vi "Streaming Xcvr (FPGA) Rx.vi"() -> ()   [LabVIEW 2016]
doc: "Acquires data from the Rx ports and streams the data to the host while receiving data from the host and generating the resulting waveform at the Tx ports of the NI USRP-294x/295x device. Use this VI as a template for the Simple NI-USRP Streaming sample project."
uses:
  <instrlib>/_niInstr/Register Bus/v1/FPGA/Public/Read Cmd Data.ctl
  SubVIs/Tx Parameters.ctl
  HOST/2954/SubVIs/Start Trigger.ctl
  SubVIs/DUC Parameters.ctl
  <instrlib>/_niInstr/DSP/v1/Shared/Public/IQ Impairments.ctl
  <instrlib>/_niInstr/DSP/v1/Shared/Public/IQ Gain.ctl
  SubVIs/Stream Control State.ctl
  SubVIs/Rx Parameters.ctl
  SubVIs/DDC Parameters.ctl
  <vilib>/Platform/TimedLoop/XDataNode/timing_clust.ctl
  <vilib>/Platform/TimedLoop/XDataNode/nitl_modes.ctl
  <vilib>/Platform/TimedLoop/XDataNode/wakeup.ctl
  <vilib>/rvi/Emulation/niFpgaProcessEmulError.vi
  <vilib>/rvi/Emulation/niFpgaSctlEmulationGetInTimedLoop.vi
  <vilib>/rvi/Emulation/niFpgaEmulationReportErrorSimple.vi
  <vilib>/rvi/Emulation/niFpgaGetClockAttributes.vi
  <vilib>/rvi/Emulation/niFpgaCriticalErrorInLSC.vi
  <vilib>/rvi/Emulation/niFpgaEmulationIsFPGAContextNoSignature.vi
  <vilib>/rvi/DataTransferAndStorage/Container/Common/niFpgaContainerGetUniqueNameForEmu.vi
  <vilib>/rvi/Memory/Memory_Emulation/niFpgaMemoryEmulationCacheClearOnFirstRun.vi
  <vilib>/rvi/Memory/Memory_Emulation/nirvimemoryEmulationManagerCache_MakeExclusive.vi
  <vilib>/rvi/Memory/Memory_Emulation/niFpgaMemoryEmulationValidateCache.vi
  <vilib>/rvi/Memory/Memory_Emulation/nirvimemoryEmulationManagerCache_InsertValue.vi
  <vilib>/Utility/error.llb/Clear Errors.vi
  <vilib>/rvi/Memory/Memory_Emulation/nirvimemoryEmulationManagerCache_ReleaseExclusive.vi
  <vilib>/rvi/Memory/Memory_Emulation/nirvimemoryEmulationManagerCache_GetValue.vi
  <vilib>/rvi/Memory/Memory_Emulation/nirvimemoryEmulationManagerCache_SetValue.vi
  <vilib>/rvi/eio/common/nirviEmuTemplateMethod_errors.vi
  <vilib>/rvi/DataTransferAndStorage/Container/Common/niFpgaContainerExecOnDevCompGetState.vi
  <vilib>/rvi/errors/niFpgaSetErrorForExecOnDevCompSimple.vi
  <vilib>/rvi/eio/common/nirviEmuReportErrorAndStop.vi
  <vilib>/rvi/FIFO/Fifo_Resource/nirvififoEmulationSetSize.vi
  <vilib>/rvi/FIFO/Fifo_Resource/nirviFifoEmulationQueueMgr.vi
  <instcachedir>/0/nirviFifoEmulationQueueMgr_E5CAEC123FF24DC58D834DCA3CDAA9B5.lvgen/nirviFifoEmulationQueueMgr_E5CAEC123FF24DC58D834DCA3CDAA9B5_004.vi
  <vilib>/rvi/FIFO/Fifo_Resource/nirvififoEmulationDetermineInputValidOut.vi
  <vilib>/rvi/FIFO/Fifo_Resource/nirvififoEmulationCreateLock.vi
  <vilib>/rvi/FIFO/Fifo_Resource/nirvififoEmulationObtainLock.vi
  <vilib>/rvi/FIFO/Fifo_Resource/nirvififoEmulationReleaseLock.vi
  <vilib>/rvi/occurrence/nirviWaitOnOccurrenceBase.vi
  <vilib>/rvi/errors/nirviReportUnexpectedCaseInternalError.vi
  <vilib>/rvi/errors/nirviReportUnexpectedCaseInternalError (U32).vi
  <vilib>/Platform/TimedLoop/XDataNode/XDataNode.xnode
  <vilib>/rvi/DataTransferAndStorage/Container/XNode/niFpgaContainer.xnode
  <vilib>/rvi/DataTransferAndStorage/Register/Emulation/niFpgaRegisterEmulation.vi
  <vilib>/eio/EIONode/EIONode.xnode
  <vilib>/rvi/DataTransferAndStorage/Register/Emulation/niFpgaRegisterEmulationRefIn.vi
  <vilib>/rvi/FIFO/Fifo_Resource/nirvififoEmulationWrite.vi
  <vilib>/Platform/TimedLoop/XDataNode/XDNodeRunTimeDep.lvlib
  <instrlib>/niUsrpRio/Config/v1/FPGA/niUsrpRio Config v1 FPGA.lvlib
  <instrlib>/_niInstr/DSP/v1/Shared/niInstr DSP v1 Shared.lvlib
  <instrlib>/_niInstr/Instruction Framework/v1/FPGA/Top Level Bus/Register Configuration/Register Configuration.lvclass
  <instrlib>/_niInstr/FIFO Register Bus/v1/FPGA/niInstr FIFO Register Bus v1 FPGA.lvclass
  <instrlib>/_niInstr/Register Bus/v1/FPGA/niInstr Register Bus v1 FPGA.lvlib
panel:
  out "F0":u32
  out "F1":u32
  out "fifo reg bus status 1":u32
  out "fifo reg bus data 1":u64
  in  "fifo reg bus ctrl 1":u32
  in  "sfp 0.core reset":bool
  in  "sfp 1.core reset":bool
  out "sfp 0.link reset":bool
  out "sfp 1.link reset":bool
  out "sfp 0.debug info":T1
  out "sfp 1.debug info":T1
  in  "rx 3.led":T2(ring)
  in  "rx 2.led":T2(ring)
  in  "rx 0.led":T2(ring)
  in  "rx 1.led":T2(ring)
  in  "tx 0.led":enum16{"None", "RF 0/TX 1", "RF 1/TX 1"}(ring)
  in  "tx 1.led":enum16{"None", "RF 0/TX 1", "RF 1/TX 1"}(ring)
  in  "rx 3.stream enable":bool
  in  "rx 2.stream enable":bool
  out "rx 3.number of iq data overflows":u64
  out "rx 2.number of iq data overflows":u64
  in  "rx 3.phase":fxp<+/-,21,0>
  in  "rx 3.frequency shift":fxp<+/-,48,0> format="%#.48g"
  in  "rx 3.impairments":T3={"inline gain I"=0.9999923706054688, "inline gain Q"=0.9999923706054688, "cross gain I"=0.0, "cross gain Q"=0.0, "pre-gain offset I"=0.0, "pre-gain offset Q"=0.0, "post-gain offset I"=0.0, "post-gain offset Q"=0.0}
  in  "rx 2.phase":fxp<+/-,21,0>
  in  "rx 2.frequency shift":fxp<+/-,48,0> format="%#.48g"
  in  "rx 2.impairments":T3={"inline gain I"=0.9999923706054688, "inline gain Q"=0.9999923706054688, "cross gain I"=0.0, "cross gain Q"=0.0, "pre-gain offset I"=0.0, "pre-gain offset Q"=0.0, "post-gain offset I"=0.0, "post-gain offset Q"=0.0}
  out "tx.status":T5={"tx.state"=enum."Idle", "tx.samples processed"=0, "tx.number of fifo underflows"=0, "tx.number of iq data overflows"=[0, 0], "tx.dsp reset done"=FALSE}
  out "rx.status":T6={"rx.state"=enum."Idle", "rx.samples processed"=0, "rx.number of fifo overflows"=0, "rx.number of iq data overflows"=[0, 0], "rx.dsp reset done"=FALSE}
  in  "rx.output sample rate":fxp<+,48,1>
  in  "rx.delay":fxp<+/-,16,0>
  in  "rx 0.frequency shift":fxp<+/-,48,0> format="%#.48g"
  in  "rx 0.phase":fxp<+/-,21,0>
  in  "rx 0.impairments":T3={"inline gain I"=0.9999923706054688, "inline gain Q"=0.9999923706054688, "cross gain I"=0.0, "cross gain Q"=0.0, "pre-gain offset I"=0.0, "pre-gain offset Q"=0.0, "post-gain offset I"=0.0, "post-gain offset Q"=0.0}
  in  "rx 1.impairments":T3={"inline gain I"=0.9999923706054688, "inline gain Q"=0.9999923706054688, "cross gain I"=0.0, "cross gain Q"=0.0, "pre-gain offset I"=0.0, "pre-gain offset Q"=0.0, "post-gain offset I"=0.0, "post-gain offset Q"=0.0}
  in  "rx 1.frequency shift":fxp<+/-,48,0> format="%#.48g"
  in  "rx 1.phase":fxp<+/-,21,0>
  in  "tx.input sample rate":fxp<+,48,1>
  in  "tx.delay":fxp<+/-,18,0>
  in  "tx 0.frequency shift":fxp<+/-,48,0> format="%#.48g"
  in  "tx 0.phase":fxp<+/-,21,0>
  in  "tx 0.impairments":T3={"inline gain I"=0.9999923706054688, "inline gain Q"=0.9999923706054688, "cross gain I"=0.0, "cross gain Q"=0.0, "pre-gain offset I"=0.0, "pre-gain offset Q"=0.0, "post-gain offset I"=0.0, "post-gain offset Q"=0.0}
  in  "tx 0.gain":T7={"gain I"=1.0, "gain Q"=1.0}
  in  "tx 1.impairments":T3={"inline gain I"=0.9999923706054688, "inline gain Q"=0.9999923706054688, "cross gain I"=0.0, "cross gain Q"=0.0, "pre-gain offset I"=0.0, "pre-gain offset Q"=0.0, "post-gain offset I"=0.0, "post-gain offset Q"=0.0}
  in  "tx 1.frequency shift":fxp<+/-,48,0> format="%#.48g"
  in  "tx 1.phase":fxp<+/-,21,0>
  in  "tx 1.gain":T7={"gain I"=1.0, "gain Q"=1.0}
  in  "rx.reset":bool=TRUE
  in  "rx.samples to acquire":u32
  in  "rx.abort":bool
  in  "tx.abort":bool
  in  "tx.reset":bool=TRUE
  in  "tx.samples to generate":u32
  in  "rx 0.stream enable":bool
  in  "rx 1.stream enable":bool
  in  "rx.trigger select":T8=enum."Immediate"
  in  "rx.software trigger":bool
  in  "rx.trigger enable":bool
  in  "tx 0.stream enable":bool
  in  "tx 1.stream enable":bool
  in  "tx.trigger select":T8=enum."Immediate"
  in  "tx.software trigger":bool
  in  "tx.trigger enable":bool
  out "rx.parameters":T9={"rx.trigger select"=enum."Software", "rx.trigger enable"=FALSE, "rx.trigger sync enable"=FALSE, "rx.stream enable"=[FALSE, FALSE, FALSE, FALSE], "rx.software trigger"=FALSE, "rx.reset"=FALSE, "rx.abort"=FALSE, "rx.samples to acquire"=0, "rx.data sink"=enum."SFP Port 0", "rx.ddc parameters"=[{"output sample rate"=0.0, "delay"=0.0, "frequency shift"=0.0, "impairments"={"inline gain I"=0.0, "inline gain Q"=0.0, "cross gain I"=0.0, "cross gain Q"=0.0, "pre-gain offset I"=0.0, "pre-gain offset Q"=0.0, "post-gain offset I"=0.0, "post-gain offset Q"=0.0}, "phase"=0.0}, {"output sample rate"=0.0, "delay"=0.0, "frequency shift"=0.0, "impairments"={"inline gain I"=0.0, "inline gain Q"=0.0, "cross gain I"=0.0, "cross gain Q"=0.0, "pre-gain offset I"=0.0, "pre-gain offset Q"=0.0, "post-gain offset I"=0.0, "post-gain offset Q"=0.0}, "phase"=0.0}, {"output sample rate"=0.0, "delay"=0.0, "frequency shift"=0.0, "impairments"={"inline gain I"=0.0, "inline gain Q"=0.0, "cross gain I"=0.0, "cross gain Q"=0.0, "pre-gain offset I"=0.0, "pre-gain offset Q"=0.0, "post-gain offset I"=0.0, "post-gain offset Q"=0.0}, "phase"=0.0}, {"output sample rate"=0.0, "delay"=0.0, "frequency shift"=0.0, "impairments"={"inline gain I"=0.0, "inline gain Q"=0.0, "cross gain I"=0.0, "cross gain Q"=0.0, "pre-gain offset I"=0.0, "pre-gain offset Q"=0.0, "post-gain offset I"=0.0, "post-gain offset Q"=0.0}, "phase"=0.0}]} {"rx.ddc parameters"."frequency shift" format="%#.48g"}
  out "rx.samples processed":u32
  out "rx.state":T4
  out "rx 0.number of iq data overflows":u64
  out "rx.number of fifo overflows":u32
  out "tx.samples processed":u32
  out "tx.number of fifo underflows":u32
  out "tx 0.number of iq data overflows":u64
  out "tx.state":T4
  out "rx.dsp reset done":bool
  out "tx.dsp reset done":bool
  out "tx 1.number of iq data overflows":u64
  out "rx 1.number of iq data overflows":u64
  out "tx.parameters":T11={"tx.trigger select"=enum."Software", "tx.trigger enable"=FALSE, "tx.trigger sync enable"=FALSE, "tx.stream enable"=[FALSE, FALSE], "tx.software trigger"=FALSE, "tx.reset"=FALSE, "tx.abort"=FALSE, "tx.samples to generate"=0, "tx.data source"=enum."SFP Port 0", "tx.duc parameters"=[{"frequency shift"=0.0, "impairments"={"inline gain I"=0.0, "inline gain Q"=0.0, "cross gain I"=0.0, "cross gain Q"=0.0, "pre-gain offset I"=0.0, "pre-gain offset Q"=0.0, "post-gain offset I"=0.0, "post-gain offset Q"=0.0}, "phase"=0.0, "input sample rate"=0.0, "gain"={"gain I"=0.0, "gain Q"=0.0}, "delay"=0.0}, {"frequency shift"=0.0, "impairments"={"inline gain I"=0.0, "inline gain Q"=0.0, "cross gain I"=0.0, "cross gain Q"=0.0, "pre-gain offset I"=0.0, "pre-gain offset Q"=0.0, "post-gain offset I"=0.0, "post-gain offset Q"=0.0}, "phase"=0.0, "input sample rate"=0.0, "gain"={"gain I"=0.0, "gain Q"=0.0}, "delay"=0.0}]} {"tx.duc parameters"."frequency shift" format="%#.48g"}
  in  "rx.trigger sync enable":bool
  in  "tx.trigger sync enable":bool
  in  "rx.data sink":enum16{"SFP Port 0", "SFP Port 1", "Host"}(ring)=enum."Host"
  in  "tx.data source":enum16{"SFP Port 0", "SFP Port 1", "Host"}(ring)=enum."Host"
  in  "RF 1/Tx/Enable":bool
  in  "RF 1/Rx/Enable":bool
  in  "RF 0/Tx/Enable":bool
  in  "RF 0/Rx/Enable":bool
  in  "reg.host read.go rcvd 0":bool
  out "reg.notify host.go 0":bool
  in  "reg.notify host.go rcvd 0":bool
  out "reg.host read.data 0":T13
  in  "reg.reset 0":bool
  # "FPGA utilization for 120 MS/s"
  # "FPGA utilization for 200 MS/s"
  # "USRP RIO Simple Streaming FPGA"
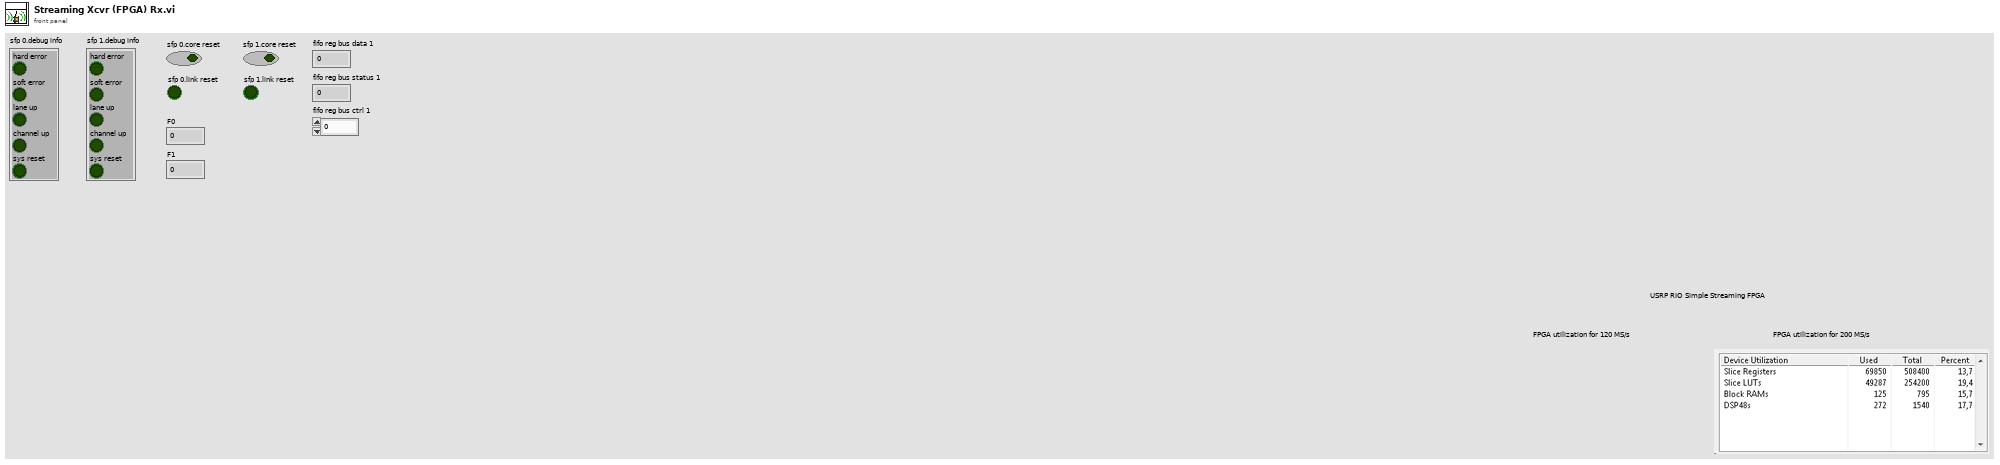
[diagram p1: front panel]
types:
  T1 = cluster{"hard error":bool, "soft error":bool, "lane up":bool, "channel up":bool, "sys reset":bool}
  T2 = enum16{"None", "RF 0/RX 1", "RF 0/RX 2", "RF 1/RX 1", "RF 1/RX 2"}
  T3 = typedef "niInstr DSP v1 Shared.lvlib/IQ Impairments.ctl" = cluster{"inline gain I":fxp<+/-,18,1>, "inline gain Q":fxp<+/-,18,1>, "cross gain I":fxp<+/-,18,1>, "cross gain Q":fxp<+/-,18,1>, "pre-gain offset I":fxp<+/-,18,1>, "pre-gain offset Q":fxp<+/-,18,1>, "post-gain offset I":fxp<+/-,18,1>, "post-gain offset Q":fxp<+/-,18,1>}
  T4 = typedef "Stream Control State.ctl" = enum16{"Idle", "Active"}
  T5 = cluster{"tx.state":T4, "tx.samples processed":u32, "tx.number of fifo underflows":u32, "tx.number of iq data overflows":u64[], "tx.dsp reset done":bool}
  T6 = cluster{"rx.state":T4, "rx.samples processed":u32, "rx.number of fifo overflows":u32, "rx.number of iq data overflows":u64[], "rx.dsp reset done":bool}
  T7 = typedef "niInstr DSP v1 Shared.lvlib/IQ Gain.ctl" = cluster{"gain I":fxp<+/-,24,3>, "gain Q":fxp<+/-,24,3>}
  T8 = typedef "Start Trigger.ctl" = enum8{"Software", "Digital Edge", "Rx Start Trigger", "Tx Start Trigger", "Immediate", "Future Time Event"}
  T9 = typedef "Rx Parameters.ctl" = cluster{"rx.trigger select":T8, "rx.trigger enable":bool, "rx.trigger sync enable":bool, "rx.stream enable":bool[], "rx.software trigger":bool, "rx.reset":bool, "rx.abort":bool, "rx.samples to acquire":u32, "rx.data sink":enum16{"SFP Port 0", "SFP Port 1", "Host"}, "rx.ddc parameters":T10[]}
  T10 = typedef "DDC Parameters.ctl" = cluster{"output sample rate":fxp<+,48,1>, "delay":fxp<+/-,16,0>, "frequency shift":fxp<+/-,48,0>, "impairments":T3, "phase":fxp<+/-,21,0>}
  T11 = typedef "Tx Parameters.ctl" = cluster{"tx.trigger select":T8, "tx.trigger enable":bool, "tx.trigger sync enable":bool, "tx.stream enable":bool[], "tx.software trigger":bool, "tx.reset":bool, "tx.abort":bool, "tx.samples to generate":u32, "tx.data source":enum16{"SFP Port 0", "SFP Port 1", "Host"}, "tx.duc parameters":T12[]}
  T12 = typedef "DUC Parameters.ctl" = cluster{"frequency shift":fxp<+/-,48,0>, "impairments":T3, "phase":fxp<+/-,21,0>, "input sample rate":fxp<+,48,1>, "gain":T7, "delay":fxp<+/-,18,0>}
  T13 = typedef "niInstr Register Bus v1 FPGA.lvlib/Read Cmd Data.ctl" = cluster{"go":bool, "data":u32}
  T14 = typedef "XDNodeRunTimeDep.lvlib/timing_clust.ctl" = cluster{"Expected End [f-1]":u64, "Actual End [f-1]":u64, "Finished Late? [f-1]":bool, "Expected End [i-1]":u64, "Actual End [i-1]":u64, "Finished Late? [i-1]":bool, "Expected Start [i]":u64, "Actual Start [i]":u64, "Expected Start [f]":u64, "Actual Start [f]":u64, "Source Name":string, "Structure Name":string, "Period":i64, "Deadline":i64, "Offset":i64, "Start":i64, "Priority":i32, "Timeout":i32, "Mode":T15, "Wakeup Reason":T16, "Error":errorcluster, "Source Type":string, "Secondary Source Type":string, "Global End Time":u64, "Global Start Time":u64, "Frame Duration":u64, "Iteration Duration":u64, "Assigned CPU":i32, "I/O Scan Engine Mode":u32}
  T15 = typedef "XDNodeRunTimeDep.lvlib/nitl_modes.ctl" = enum32{"No Change", "Process missed periods, maintain original phase", "Discard missed periods, maintain original phase", "Process missed periods, ignore original phase", "Discard missed periods, ignore original phase"}
  T16 = typedef "XDNodeRunTimeDep.lvlib/wakeup.ctl" = enum32{"Normal", "Aborted", "Asynchronous wakeup", "Timing source error", "Timed loop error", "Timeout"}
  T17 = cluster{"tx 0.led":enum16{"None", "RF 0/TX 1", "RF 1/TX 1"}, "tx 1.led ":enum16{"None", "RF 0/TX 1", "RF 1/TX 1"}}
  T18 = cluster{"rx 0.led":enum16{"None", "RF 0/RX 1", "RF 0/RX 2", "RF 1/RX 1", "RF 1/RX 2"}, "rx 1.led":enum16{"None", "RF 0/RX 1", "RF 0/RX 2", "RF 1/RX 1", "RF 1/RX 2"}}
  T19 = cluster{"DAC FIFO Reset":refnum<k21>, "RF 0 Rx Swap IQ":refnum<k21>, "RF 0 Rx Negate I":refnum<k21>, "RF 0 Rx Negate Q":refnum<k21>, "RF 0 Rx Data Valid":refnum<k21>, "RF 0 Rx Data Ever Invalid":refnum<k21>, "clear RF 0 Rx Data Ever Invalid":refnum<k21>, "RF 0 Tx Swap IQ":refnum<k21>, "RF 0 Tx Negate I":refnum<k21>, "RF 0 Tx Negate Q":refnum<k21>, "RF 1 Rx Swap IQ":refnum<k21>, "RF 1 Rx Negate I":refnum<k21>, "RF 1 Rx Negate Q":refnum<k21>, "RF 1 Rx Data Valid":refnum<k21>, "RF 1 Rx Data Ever Invalid":refnum<k21>, "clear RF 1 Rx Data Ever Invalid":refnum<k21>, "RF 1 Tx Swap IQ":refnum<k21>, "RF 1 Tx Negate I":refnum<k21>, "RF 1 Tx Negate Q":refnum<k21>}
  T20 = typedef "niUsrpRio Synchronization v1 FPGA.lvlib/Resources.ctl" = cluster{"master":refnum<k21>, "meas.enable":refnum<k21>, "meas.ready":refnum<k21>, "meas.reset":refnum<k21>, "meas.arm":refnum<k21>, "meas.valid":refnum<k21>, "meas.value":refnum<k21>, "meas.oversample factor":refnum<k21>, "cptr":refnum<k21>, "cptr.adjust":refnum<k21>, "cptr.period":refnum<k21>}
  T21 = typedef "niUsrpRio Time v1 FPGA.lvlib/Time Resources.ctl" = cluster{"reset":refnum<k21>, "time":refnum<k21>, "time.previous cptr":refnum<k21>, "new time":refnum<k21>, "new time.when":refnum<k21>, "new time.set":refnum<k21>, "which edge of ref":refnum<k21>, "pps source":refnum<k21>, "internal pps period":refnum<k21>}
  T22 = typedef "niUsrpRio Time v1 FPGA.lvlib/Future Event Resources.ctl" = cluster{"reset":refnum<k21>, "future event.time":refnum<k21>, "future event.ready":refnum<k21>, "future event.set":refnum<k21>, "future event.clear":refnum<k21>, "future event.set in past":refnum<k21>}
  T23 = cluster{"time.resources":T21, "future event.resources":T22, "future event.resources":T22, "future event.resources":T22}
  T24 = cluster{"port clock":refnum<k21>, "TX niInstr AXI4-Stream Reader FXP64x1 v1 FPGA out":refnum<class "niInstr AXI4-Stream Writer FXP64x1 v1 FPGA.lvclass">, "RX niInstr AXI4-Stream Reader FXP64x1 v1 FPGA out":refnum<class "niInstr AXI4-Stream Reader FXP64x1 v1 FPGA.lvclass">, "Port 0 Debug CLIP Resources":cluster{"Hard Error":refnum<k21>, "Soft Error":refnum<k21>, "Lane Up":refnum<k21>, "Channel Up":refnum<k21>, "Sys Reset":refnum<k21>}, "debug info":refnum<k21>}
  T25 = cluster{"port clock":refnum<k21>, "TX niInstr AXI4-Stream Reader FXP64x1 v1 FPGA out":refnum<class "niInstr AXI4-Stream Writer FXP64x1 v1 FPGA.lvclass">, "RX niInstr AXI4-Stream Reader FXP64x1 v1 FPGA out":refnum<class "niInstr AXI4-Stream Reader FXP64x1 v1 FPGA.lvclass">, "Port 1 Debug CLIP Resources":cluster{"Hard Error":refnum<k21>, "Soft Error":refnum<k21>, "Lane Up":refnum<k21>, "Channel Up":refnum<k21>, "Sys Reset":refnum<k21>}, "debug info":refnum<k21>}
  T26 = cluster{"rx.trigger select":T8, "rx.trigger enable":bool, "rx.trigger sync enable":bool, bool[], "rx.software trigger":bool, "rx.reset":bool, "rx.abort":bool, "rx.samples to acquire":u32, "rx.data sink":enum16{"SFP Port 0", "SFP Port 1", "Host"}, T10[]}
  T27 = cluster{"tx.trigger select":T8, "tx.trigger enable":bool, "tx.trigger sync enable":bool, bool[], "tx.software trigger":bool, "tx.reset":bool, "tx.abort":bool, "tx.samples to generate":u32, "tx.data source":enum16{"SFP Port 0", "SFP Port 1", "Host"}, T12[]}
  T28 = typedef "niInstr Register Bus v1 FPGA.lvlib/Register Instruction.ctl" = cluster{"subsystem":u8, "address":u16, "data":u32, "valid":bool, "read":bool}
  T29 = typedef "niInstr Register Bus v1 FPGA.lvlib/Read Completion.ctl" = cluster{"data":u32, "valid":bool}
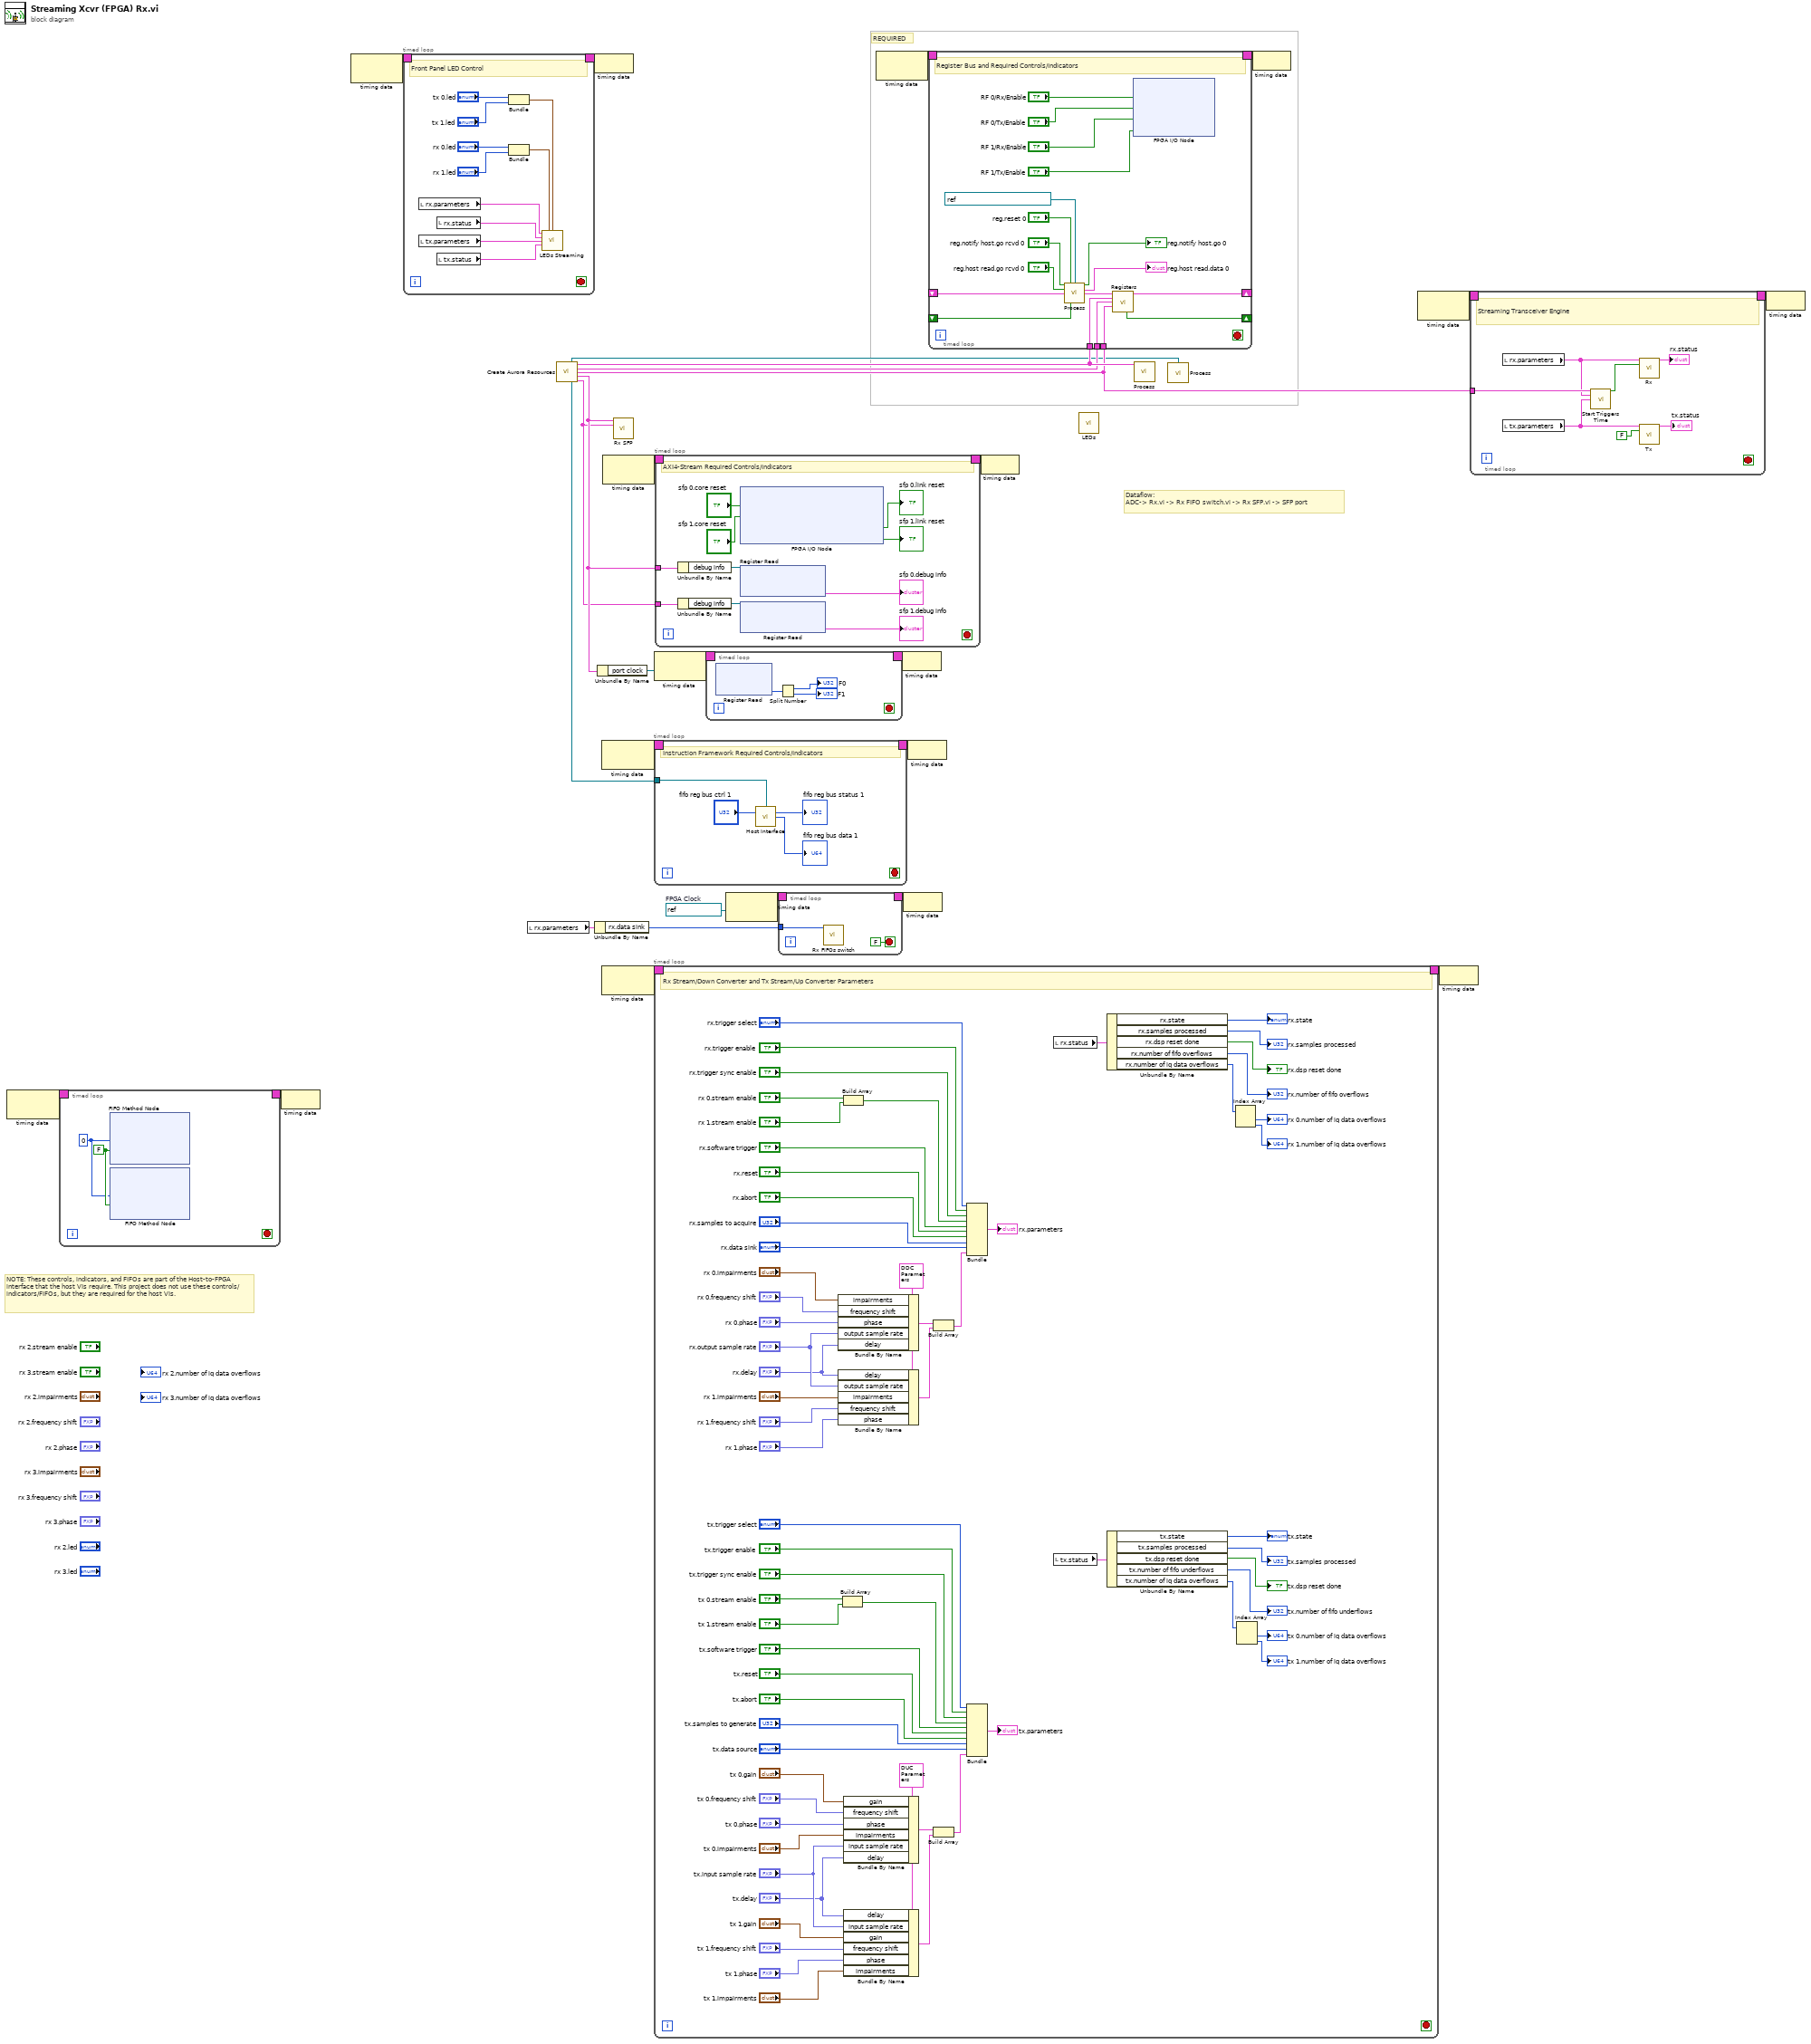
[diagram p0: block diagram]
diagram:
  w3 = refnum<k21> "Data Clock"  # FPGA Clock
  # "Dataflow:\nADC-> Rx.vi -> Rx FIFO switch.vi -> Rx SFP.vi -> SFP port"
  # "NOTE: These controls, indicators, and FIFOs are part of the Host-to-FPGA interface that the host VIs require. This project does not use these controls/indicators/FIFOs, but they are required for the host VIs."
  # "REQUIRED"
  n1 = node-c288() -> (w2:T14)  [unwired: 1 in]
  n2 = timed-loop {
    timing: w2 -> [_]
    timing-out: [_] -> w1
    stop <- _ stop-if-true
    w30 = u32 0 ("Element")
    w31 = FALSE ("Input Valid")
    n3 = xnode ("FIFO Method Node")("Element"=w30, "Input Valid"=w31) -> ()  [unwired: 1 in, 2 out]
    n4 = xnode ("FIFO Method Node")("Element"=w30, "Input Valid"=w31) -> ()  [unwired: 1 in, 2 out]
  }
  n5 = node-c288(w1) -> ()
  n6 = node-c288() -> (w23:T14)  [unwired: 1 in]
  n7 = timed-loop {
    timing: w23 -> [_]
    timing-out: [_] -> w22
    stop <- _ stop-if-true
    # "Front Panel LED Control"
    n8 = local read "rx.parameters"() -> (w37:T9)
    n9 = local read "tx.parameters"() -> (w35:T11)
    n10 = local read "rx.status"() -> (w36:T6)
    n11 = local read "tx.status"() -> (w34:T5)
    n12 = Bundle("tx 0.led"="tx 0.led", "tx 1.led"="tx 1.led") -> (w38:T17)  [unwired: 1 in]
    n13 = Bundle("rx 0.led"="rx 0.led", "rx 1.led"="rx 1.led") -> (w39:T18)  [unwired: 1 in]
    n14 = call "LEDs Streaming.vi"("rx.parameters"=w37, "rx.leds"=w39, "tx.leds"=w38, "rx.status"=w36, "tx.parameters"=w35, "tx.status"=w34) -> ()  [unwired: 10 in]
  }
  n15 = local read "rx.parameters"() -> (w10:T9)
  n16 = call "Create Aurora Resources.vi"() -> ("framework.resources"=w18:refnum<class "Register Configuration.lvclass">, "config.resources"=w21:T19, "sync.resources"=w20:T20, "time.resources"=w19:T23, "sfp 0.resources"=w7:T24, "producer.resources"=w8:refnum<class "niInstr FIFO Register Bus v1 FPGA.lvclass">, "sfp 1.resources"=w6:T25)  [unwired: 9 in]
  n17 = node-c288(w22) -> ()
  n18 = Unbundle By Name(w10) -> ("rx.data sink"=w9:enum16{"SFP Port 0", "SFP Port 1", "Host"})
  n19 = Unbundle By Name(w7) -> ("port clock"=w11:refnum<k21>)
  n20 = node-c288() -> (w15:T14)  [unwired: 1 in]
  n21 = node-c288() -> (w25:T14)  [unwired: 1 in]
  n22 = node-c288() -> (w17:T14)  [unwired: 1 in]
  n23 = call "Rx SFP.vi"("sfp 0.resources"=w7, "sfp 1.resources"=w6) -> ()  [unwired: 14 in]
  n24 = node-c288(w11) -> (w13:T14)
  n25 = timed-loop {
    timing: w15 -> [_]
    timing-out: [_] -> w14
    tunnel: w8 -> [w49]
    stop <- _ stop-if-true
    # "Instruction Framework Required Controls/Indicators"
    n26 = call <instrlib>:"Host Interface.vi"("fifo register bus"=w49, "fifo reg bus ctrl 0"="fifo reg bus ctrl 1") -> ("fifo reg bus status 0"=→"fifo reg bus status 1":u32, "fifo reg bus data 0"=→"fifo reg bus data 1":u64)  [unwired: 12 in]
  }
  n27 = timed-loop {
    timing: w25 -> [_]
    timing-out: [_] -> w24
    stop <- _ stop-if-true
    w106 = T12 {"frequency shift"=0.0, "impairments"={"inline gain I"=0.9999923706054688, "inline gain Q"=0.9999923706054688, "cross gain I"=0.0, "cross gain Q"=0.0, "pre-gain offset I"=0.0, "pre-gain offset Q"=0.0, "post-gain offset I"=0.0, "post-gain offset Q"=0.0}, "phase"=0.0, "input sample rate"=0.0, "gain"={"gain I"=1.0, "gain Q"=1.0}, "delay"=0.0} ("DUC Parameters")
    w117 = T10 {"output sample rate"=1.0, "delay"=0.0, "frequency shift"=0.0, "impairments"={"inline gain I"=0.9999923706054688, "inline gain Q"=0.9999923706054688, "cross gain I"=0.0, "cross gain Q"=0.0, "pre-gain offset I"=0.0, "pre-gain offset Q"=0.0, "post-gain offset I"=0.0, "post-gain offset Q"=0.0}, "phase"=0.0} ("DDC Parameters")
    # "Rx Stream/Down Converter and Tx Stream/Up Converter Parameters"
    n28 = Bundle By Name(cluster=w117, "impairments"="rx 0.impairments", "frequency shift"="rx 0.frequency shift", "phase"="rx 0.phase", "output sample rate"="rx.output sample rate", "delay"="rx.delay") -> (w115:T10)
    n29 = Bundle By Name(cluster=w117, "delay"="rx.delay", "output sample rate"="rx.output sample rate", "impairments"="rx 1.impairments", "frequency shift"="rx 1.frequency shift", "phase"="rx 1.phase") -> (w116:T10)
    n30 = Build Array("tx 0.stream enable", "tx 1.stream enable") -> (w63:bool[])
    n31 = Build Array("rx 0.stream enable", "rx 1.stream enable") -> (w65:bool[])
    n32 = Bundle By Name(cluster=w106, "gain"="tx 0.gain", "frequency shift"="tx 0.frequency shift", "phase"="tx 0.phase", "impairments"="tx 0.impairments", "input sample rate"="tx.input sample rate", "delay"="tx.delay") -> (w104:T12)
    n33 = Bundle By Name(cluster=w106, "delay"="tx.delay", "input sample rate"="tx.input sample rate", "gain"="tx 1.gain", "frequency shift"="tx 1.frequency shift", "phase"="tx 1.phase", "impairments"="tx 1.impairments") -> (w105:T12)
    n34 = Build Array(w115, w116) -> (w86:T10[])
    n35 = Build Array(w104, w105) -> (w84:T12[])
    n36 = Bundle("rx.trigger select"="rx.trigger select", "rx.trigger enable"="rx.trigger enable", "rx.trigger sync enable"="rx.trigger sync enable", w65, "rx.software trigger"="rx.software trigger", "rx.reset"="rx.reset", "rx.abort"="rx.abort", "rx.samples to acquire"="rx.samples to acquire", "rx.data sink"="rx.data sink", w86) -> (→"rx.parameters":T26)  [unwired: 1 in]
    n37 = Bundle("tx.trigger select"="tx.trigger select", "tx.trigger enable"="tx.trigger enable", "tx.trigger sync enable"="tx.trigger sync enable", w63, "tx.software trigger"="tx.software trigger", "tx.reset"="tx.reset", "tx.abort"="tx.abort", "tx.samples to generate"="tx.samples to generate", "tx.data source"="tx.data source", w84) -> (→"tx.parameters":T27)  [unwired: 1 in]
    n38 = local read "rx.status"() -> (w77:T6)
    n39 = local read "tx.status"() -> (w74:T5)
    n40 = Unbundle By Name(w77) -> ("rx.state"=→"rx.state":T4, "rx.samples processed"=→"rx.samples processed":u32, "rx.dsp reset done"=→"rx.dsp reset done":bool, "rx.number of fifo overflows"=→"rx.number of fifo overflows":u32, "rx.number of iq data overflows"=w54:u64[])
    n41 = Unbundle By Name(w74) -> ("tx.state"=→"tx.state":T4, "tx.samples processed"=→"tx.samples processed":u32, "tx.dsp reset done"=→"tx.dsp reset done":bool, "tx.number of fifo underflows"=→"tx.number of fifo underflows":u32, "tx.number of iq data overflows"=w57:u64[])
    n42 = Index Array(array=w54) -> (element #1=→"rx 0.number of iq data overflows":u64, element #2=→"rx 1.number of iq data overflows":u64)  [unwired: 2 in]
    n43 = Index Array(array=w57) -> (element #1=→"tx 0.number of iq data overflows":u64, element #2=→"tx 1.number of iq data overflows":u64)  [unwired: 2 in]
  }
  n44 = timed-loop {
    timing: w17 -> [_]
    timing-out: [_] -> w16
    tunnel: w7 -> [w125]
    tunnel: w6 -> [w124]
    stop <- _ stop-if-true
    # "AXI4-Stream Required Controls/Indicators"
    n45 = Unbundle By Name(w125) -> ("debug info"=w123:refnum<k21>)
    n46 = Unbundle By Name(w124) -> ("debug info"=w122:refnum<k21>)
    n47 = xnode "FPGA I/O Node"("MGT Socket\\dPort0CoreReset"="sfp 0.core reset", "MGT Socket\\dPort1CoreReset"="sfp 1.core reset") -> ("MGT Socket\\dPort0LinkResetOut"=→"sfp 0.link reset":bool, "MGT Socket\\dPort1LinkResetOut"=→"sfp 1.link reset":bool)  [unwired: 4 in, 4 out]
    n48 = xnode ("Register Read")("Register In"=w123) -> ("Data"=→"sfp 0.debug info":T1)  [unwired: 1 out]
    n49 = xnode ("Register Read")("Register In"=w122) -> ("Data"=→"sfp 1.debug info":T1)  [unwired: 1 out]
  }
  n50 = timed-loop {
    timing: w13 -> [_]
    timing-out: [_] -> w12
    stop <- _ stop-if-true
    n51 = xnode ("Register Read")() -> ("Data"=w134:u64)  [unwired: 1 in, 1 out]
    n52 = Split Number(x=w134) -> (hi(x)=→"F0":u32, lo(x)=→"F1":u32)
  }
  n53 = node-c288(w3) -> (w5:T14)
  n54 = timed-loop {
    timing: w5 -> [_]
    timing-out: [_] -> w4
    tunnel: w9 -> [w138]
    stop <- FALSE stop-if-true
    n55 = call "Rx FIFOs switch.vi"("rx.data sink"=w138) -> ()  [unwired: 15 in]
  }
  n56 = node-c288() -> (w29:T14)  [unwired: 1 in]
  n57 = node-c288(w12) -> ()
  n58 = node-c288(w4) -> ()
  n59 = node-c288(w14) -> ()
  n60 = timed-loop "Register Bus and Required Controls/Indicators" {
    timing: w29 -> [_]
    timing-out: [_] -> w28
    tunnel: w21 -> [w153]
    tunnel: w20 -> [w152]
    tunnel: w19 -> [w151]
    shift-right: [w150] -> _
    shift-left: _ -> [w149]
    shift-right: [w141] -> _
    shift-left: _ -> [w142]
    stop <- _ stop-if-true
    # "Register Bus and Required Controls/Indicators"
    n61 = call <instrlib>:"Process.vi"("reg.notify host.go rcvd"="reg.notify host.go rcvd 0", "reg.reset"="reg.reset 0", "reg.host instruction fifo"=refnum<k21> "reg.host instruction fifo 0", "reg.host read.go rcvd"="reg.host read.go rcvd 0", "read completion"=w142, "ready for output"=w149) -> ("reg.notify host.go"=→"reg.notify host.go 0":bool, "reg.host read.data"=→"reg.host read.data 0":T13, "register instruction"=w154:T28)  [unwired: 7 in]
    n62 = call "Registers.vi"("register instruction"=w154, "config.resources"=w153, "sync.resources"=w152, "time.resources"=w151) -> ("read completion out"=w141:T29, "ready for input"=w150:bool)  [unwired: 10 in]
    n63 = xnode ("FPGA I/O Node")("RF 0/Rx/Enable"="RF 0/Rx/Enable", "RF 0/Tx/Enable"="RF 0/Tx/Enable", "RF 1/Rx/Enable"="RF 1/Rx/Enable", "RF 1/Tx/Enable"="RF 1/Tx/Enable") -> ()  [unwired: 4 in, 4 out]
  }
  n64 = node-c288(w16) -> ()
  n65 = call "LEDs.vi"() -> ()  [unwired: 1 in]
  n66 = call <instrlib>:"Process.vi"("resources"=w21) -> ()  [unwired: 15 in]
  n67 = call <instrlib>:"Process.vi"("register configuration"=w18) -> ()  [unwired: 15 in]
  n68 = node-c288(w28) -> ()
  n69 = node-c288() -> (w27:T14)  [unwired: 1 in]
  n70 = node-c288(w24) -> ()
  n71 = timed-loop "Streaming Transceiver Engine" {
    timing: w27 -> [_]
    timing-out: [_] -> w26
    tunnel: w19 -> [w167]
    stop <- _ stop-if-true
    # "Streaming Transceiver Engine"
    n72 = local read "rx.parameters"() -> (w165:T9)
    n73 = local read "tx.parameters"() -> (w166:T11)
    n74 = call "Start Triggers Time.vi"("time.resources"=w167, "rx.parameters"=w165, "tx.parameters"=w166) -> ("rx.start trigger"=w161:bool)  [unwired: 11 in, 1 out]
    n75 = call "Rx.vi"("rx.parameters"=w165, "rx.start trigger"=w161) -> ("rx.status"=→"rx.status":T6)  [unwired: 13 in]
    n76 = call "Tx.vi"("tx.parameters"=w166, "tx.start trigger"=FALSE) -> ("tx.status"=→"tx.status":T5)  [unwired: 13 in]
  }
  n77 = node-c288(w26) -> ()
